vi "5668 Plot Spectrum.vi"(8 "error in":errorcluster, 10 "Config Data in":T1={" Start Carrier Frequency (Hz)"=4000000000.0, "Stop Carrier Frequency (Hz)"=6000000000.0, "Resolution Bandwidth (Hz)"=10000.0, "Overlap"=enum."Overlap"} {"Resolution Bandwidth (Hz)" format="%#_6p"; "Stop Carrier Frequency (Hz)" format="%#_6p"; "Start Carrier Frequency (Hz)" format="%#_6p"}, 11 "Data":waveform(cdb)[](array[waveform])) -> (0 "error out":errorcluster, 3 "Power Spectrum":cluster{"f0":dbl, "df":dbl, "magnitude":dbl[]})   [LabVIEW 2017]
uses:
  Config Data.ctl
  <vilib>/Analysis/4window.llb/windowTd.ctl
  <vilib>/measure/maspectr.llb/FFT Power Spectrum and PSD for 1 Chan (CDB).vi
  <vilib>/Analysis/NI_AALPro.lvlib
  <vilib>/measure/NI_MAPro.lvlib
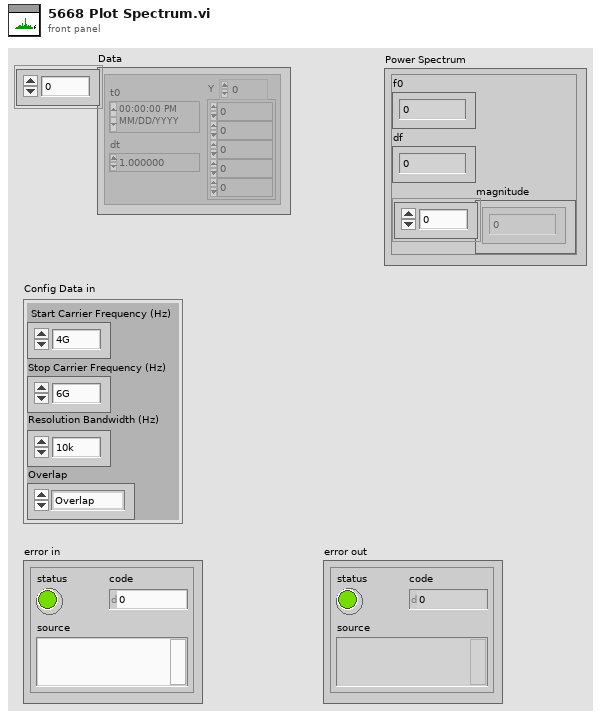
[diagram p1: front panel]
types:
  T1 = typedef "Config Data.ctl" = cluster{" Start Carrier Frequency (Hz)":dbl, "Stop Carrier Frequency (Hz)":dbl, "Resolution Bandwidth (Hz)":dbl, "Overlap":enum16{"No Overlap", "Overlap"}}
  T2 = typedef "NI_AALPro.lvlib/windowTd.ctl" = u32
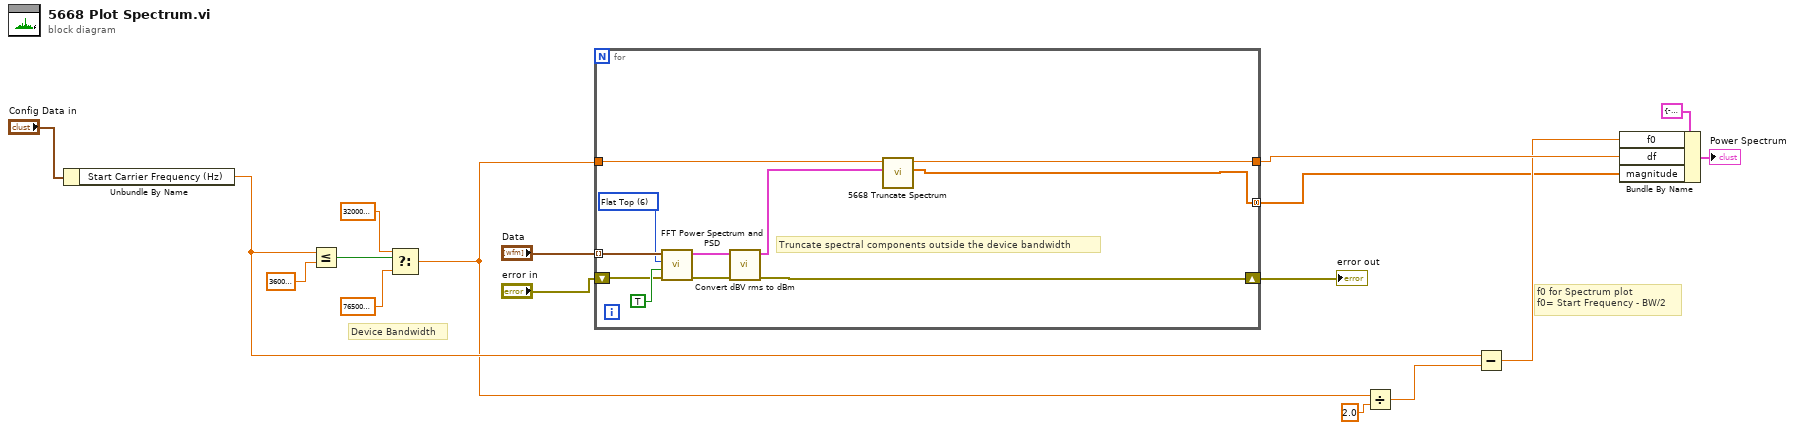
[diagram p0: block diagram]
diagram:
  # "f0 for Spectrum plot\nf0= Start Frequency - BW/2"
  # "Device Bandwidth"
  n1 = Unbundle By Name("Config Data in") -> ("Start Carrier Frequency (Hz)"=w2:dbl)
  n2 = Less Or Equal?(x=w2, y=3600000000.0) -> (x <= y?=w3:bool)
  n3 = Select(t=320000000.0 ("y"), s=w3, f=765000000.0 ("y")) -> (s? t:f=w1:dbl)
  n4 = for {
    tunnel: "Data" -> [w27] mode=indexing
    shift-right: [w23] -> w17
    shift-left: "error in" -> [w26]
    tunnel: w1 -> [w20]
    tunnel: [w19] -> w6 mode=concatenating
    tunnel: [w18] -> w8
    w22 = T2 6 items=["Rectangle"=0, "Hanning"=1, "Hamming"=2, "Blackman-Harris"=3, "Exact Blackman"=4, "Blackman"=5, "Flat Top"=6, "4 Term B-Harris "=7, "7 Term B-Harris"=8, "Low Sidelobe"=9, "Blackman Nuttall"=11, "Triangle"=30, "Bartlett-Hanning"=31, "Bohman"=32, "Parzen"=33, "Welch"=34, "Kaiser"=60, "Dolph-Chebyshev"=61, "Gaussian"=62] ("window")
    # "Truncate spectral components outside the device bandwidth"
    n5 = call-poly <vilib>:"FFT Power Spectrum and PSD.vi"("error in (no error)"=w26, "dB On (F)"=TRUE, "window"=w22, "time signal"=w27) -> ("error out"=w24:errorcluster, "Power Spectrum / PSD"=w25:cluster{"f0":dbl, "df":dbl, "magnitude":dbl[]})  [unwired: 4 in, 2 out]
    n6 = call "Convert dBV rms to dBm.vi"("error in (no error)"=w24, "Power Spectrum / PSD (dBV rms)"=w25) -> ("error out"=w23:errorcluster, "Power Spectrum / PSD (dBm)"=w21:cluster{"f0":dbl, "df":dbl, "magnitude":dbl[]})  [unwired: 8 in]
    n7 = call "5668 Truncate Spectrum.vi"("Power Spectrum / PSD (dBm)"=w21, "y"=w20) -> ("Array"=w19:dbl[], "df"=w18:dbl)  [unwired: 8 in]
  }
  "error out" <- w17
  n8 = Divide(x=w1, y=2.0) -> (x/y=w13:dbl)
  n9 = Subtract(x=w2, y=w13) -> (x-y=w7:dbl)
  n10 = Bundle By Name(cluster=cluster{"f0":dbl, "df":dbl, "magnitude":dbl[]} {"f0"=-250000000.0, "df"=10000.0, "magnitude"=array[50000 elements]} ("Array 2"), "f0"=w7, "df"=w8, "magnitude"=w6) -> (→"Power Spectrum":cluster{"f0":dbl, "df":dbl, "magnitude":dbl[]})
